vi "Reading buffer basetimestamp.vi"(8 "错误输入":errorcluster, 10 "缓冲区名称":string(combo), 11 "VISA资源名称":refnum<visa-resource-name>) -> (0 "错误输出":errorcluster, 2 "时间标识":timestamp, 3 "VISA资源名称输出":refnum<visa-resource-name>)   [LabVIEW 2020]
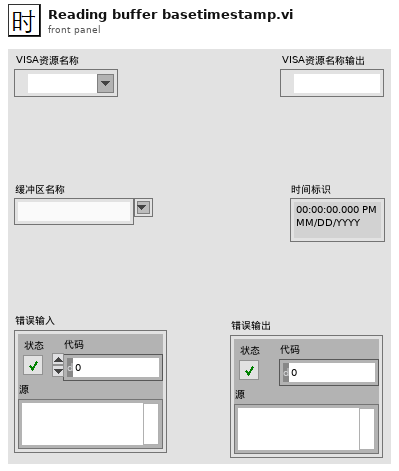
[diagram p1: front panel]
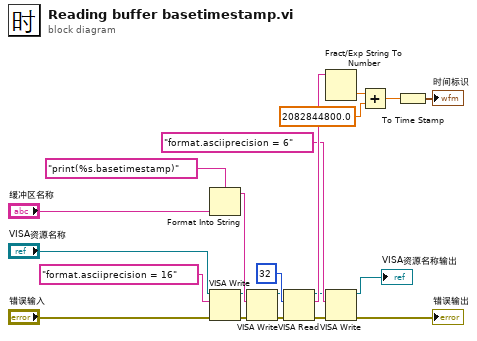
[diagram p0: block diagram]
diagram:
  n1 = Format Into String(format string="print(%s.basetimestamp)" ("格式字符串"), "缓冲区名称") -> (resulting string=w12:string)  [unwired: 2 in, 1 out]
  n2 = VISA Write(VISA resource name="VISA资源名称", write buffer="format.asciiprecision = 16" ("格式字符串"), error in (no error)="错误输入") -> (VISA resource name out=w8:refnum<visa-resource-name>, error out=w7:errorcluster)  [unwired: 1 out]
  n3 = VISA Write(VISA resource name=w8, write buffer=w12, error in (no error)=w7) -> (VISA resource name out=w6:refnum<visa-resource-name>, error out=w5:errorcluster)  [unwired: 1 out]
  n4 = VISA Read(VISA resource name=w6, byte count=u32 32 ("字节总数"), error in (no error)=w5) -> (VISA resource name out=w4:refnum<visa-resource-name>, read buffer=w15:string, error out=w3:errorcluster)  [unwired: 1 out]
  n5 = Fract/Exp String To Number(string=w15) -> (number=w13:dbl)  [unwired: 3 in, 1 out]
  n6 = VISA Write(VISA resource name=w4, write buffer="format.asciiprecision = 6" ("格式字符串"), error in (no error)=w3) -> (VISA resource name out=→"VISA资源名称输出":refnum<visa-resource-name>, error out=→"错误输出":errorcluster)  [unwired: 1 out]
  n7 = Add(x=w13, y=2082844800.0 ("x-y")) -> (x+y=w11:dbl)
  n8 = To Time Stamp(1:w11) -> (0:→"时间标识":timestamp)
